vi "mxwScript_API_Option_WireRoutingParameters.vi"(8 "error in (no error)":errorcluster, 10 "routingAlgorithm":T2=enum."AI", 11 "options in":T1[](array[typedef])) -> (0 "error out":errorcluster, 3 "options out":T1[](array[typedef]))   [LabVIEW 2017]
uses:
  codeGenAPISupport.llb/cgAPI_mxwScript_Wire_RoutingAlgorithm.ctl
  codeGenAPISupport.llb/cgAPI_mxwScript_OptionData.ctl
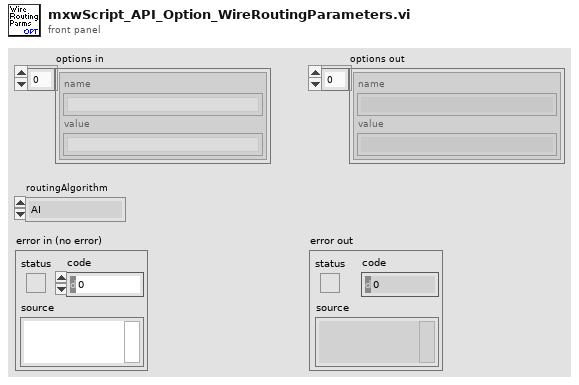
[diagram p1: front panel]
types:
  T1 = typedef "cgAPI_mxwScript_OptionData.ctl" = cluster{"name":string, "value":string}
  T2 = typedef "cgAPI_mxwScript_Wire_RoutingAlgorithm.ctl" = enum16{"None", "LV", "AI"}
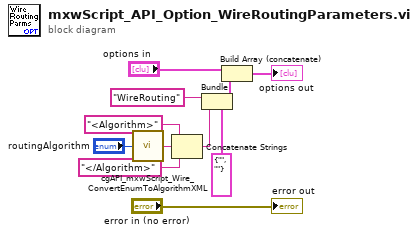
[diagram p0: block diagram]
diagram:
  n1 = call "cgAPI_mxwScript_Wire_ConvertEnumToAlgorithmXML.vi"("routingAlgorithm"="routingAlgorithm") -> ("XML out"=w2:string)  [unwired: 4 out]
  n2 = Concatenate Strings("<Algorithm>", w2, "</Algorithm>") -> (w4:string)
  n3 = Bundle(cluster=T1 {"name"="", "value"=""} ("optionData"), "name"="WireRouting", "value"=w4) -> (w9:T1)
  n4 = Build Array (concatenate)("options in", w9) -> (→"options out":T1[])
  "error out" <- "error in (no error)"
